vi "GEN2_Set_Posi.vi"(6 "Tolerance":dbl, 7 "ID":u8, 8 "error in (no error)":errorcluster, 10 "Expected Theta":dbl, 11 "VISA Refnum in":refnum<visa-resource-name>) -> (0 "error out":errorcluster, 3 "VISA Refnum out":refnum<visa-resource-name>)   [LabVIEW 2016, in "GEN_2.lvlib"]
uses:
  GEN_2.lvlib
  GEN2_Instructions.ctl
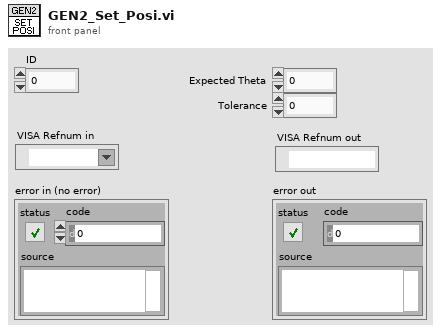
[diagram p1: front panel]
types:
  T1 = enum16{"big-endian, network order", "native, host order", "little-endian"}
  T2 = typedef "GEN_2.lvlib/GEN2_Instructions.ctl" = u8
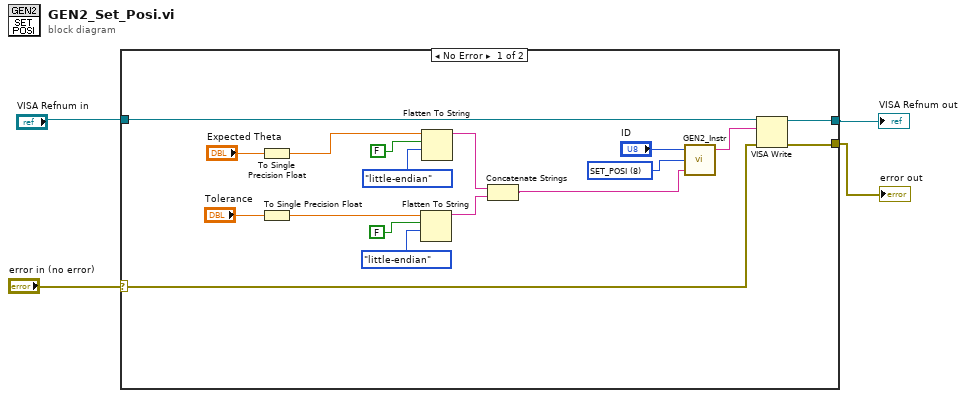
[diagram p0: block diagram]
diagram:
  n1 = case shown="No Error" "error in (no error)" {
    selector: "error in (no error)" -> [w10 w24]
    tunnel: [w21 w23] -> w4
    tunnel: [w20 w24] -> w3
    tunnel: "VISA Refnum in" -> [w17 w23]
    frame No Error {
      w16 = T2 8 items=["PING"=1, "READ_STAT"=2, "WRITE_STAT"=3, "READ_CONFIG"=4, "WRITE_CONFIG"=5, "SAVE_CONFIG"=6, "SET_POSI"=8, "BULK_STAT"=18] ("Instruction")
      n2 = To Single Precision Float(number="Expected Theta") -> (single precision float=w5:sgl)
      n3 = To Single Precision Float(number="Tolerance") -> (single precision float=w6:sgl)
      n4 = Flatten To String(anything=w6, prepend array or string size? (T)=FALSE, byte order (0:big-endian, network order)=T1."little-endian") -> (data string=w9:string)  [unwired: 1 in, 2 out]
      n5 = Flatten To String(anything=w5, prepend array or string size? (T)=FALSE, byte order (0:big-endian, network order)=T1."little-endian") -> (data string=w13:string)  [unwired: 1 in, 2 out]
      n6 = Concatenate Strings(w13, w9) -> (w22:string)
      n7 = call "GEN2_Instr.vi"("Parameter"=w22, "Instruction"=w16, "ID"="ID") -> ("Output"=w19:string)  [unwired: 2 in]
      n8 = VISA Write(VISA resource name=w17, write buffer=w19, error in (no error)=w10) -> (VISA resource name out=w21:refnum<visa-resource-name>, error out=w20:errorcluster)  [unwired: 1 out]
    }
    frame Error {
    }
  }
  "VISA Refnum out" <- w4
  "error out" <- w3
